vi "demoMode.vi"(8 "error in (no error)":errorcluster, 11 "Pod Drive in":refnum<class "Drive.lvclass">) -> (0 "error out":errorcluster, 3 "Pod Drive out":refnum<class "Drive.lvclass">)   [LabVIEW 2019, in "DriveOld.lvlib" / "Drive.lvclass"]
doc: "This VI puts the robot into demo mode. This will reduce the amount of power making the robot slower and safer."
uses:
  Drive.lvclass
  <vilib>/Rock Robotics/SystemInterfaces/DIO/FPGA_DIOChannel.ctl
  Drive.lvclass/Drive.ctl
  <vilib>/Rock Robotics/Network Tables/NT Write Boolean.vi
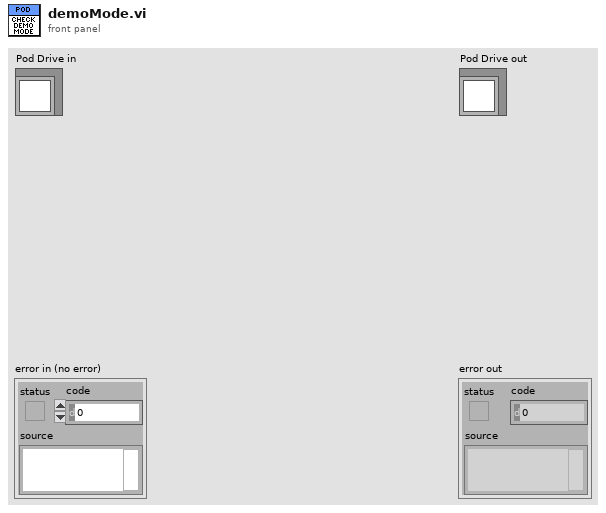
[diagram p1: front panel]
types:
  T1 = typedef "FPGA_DIOChannel.ctl" = enum8{"DIO 0", "DIO 1", "DIO 2", "DIO 3", "DIO 4", "DIO 5", "DIO 6", "DIO 7", "DIO 8", "DIO 9", "DIO MXP 0", "DIO MXP 1", "DIO MXP 2", "DIO MXP 3", "DIO MXP 4", "DIO MXP 5", "DIO MXP 6", "DIO MXP 7", "DIO MXP 8", "DIO MXP 9", "DIO MXP 10", "DIO MXP 11", "DIO MXP 12", "DIO MXP 13", "DIO MXP 14", "DIO MXP 15", "SPI Port CS1", "SPI Port CS2", "SPI Port CS3", "SPI Port MISO", "SPI Port MOSI", "Invalid"}
  T2 = typedef "WPI_DigitalInputDevRef.ctl" = cluster{"DevStatus":errorcluster, "DIO Channel":T1}
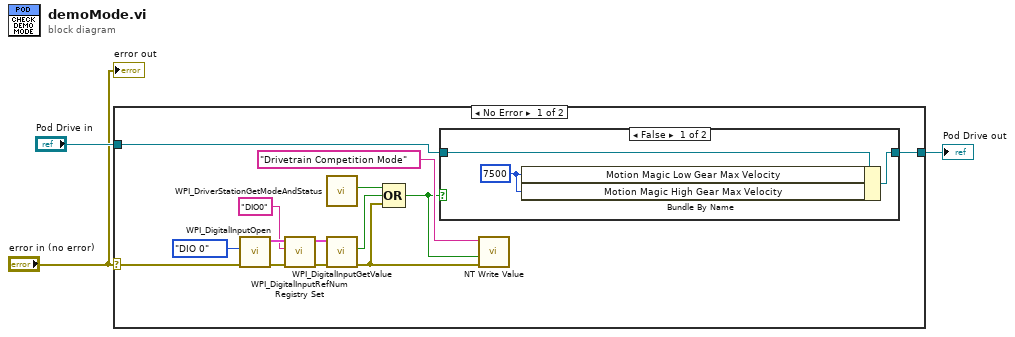
[diagram p0: block diagram]
diagram:
  n1 = case shown="No Error" "error in (no error)" {
    selector: "error in (no error)" -> [w5 _]
    tunnel: [w6 w22] -> w3
    tunnel: "Pod Drive in" -> [w7 w22]
    frame No Error {
      n2 = call <vilib>:"WPI_DigitalInputOpen.vi"("error in (no error)"=w5, "DIO Channel"=FPGA_DIOChannel."DIO 0") -> ("error out"=w16:errorcluster, "DigitalInputDevRef"=w15:T2)  [unwired: 8 in]
      n3 = call <vilib>:"WPI_DigitalInputRefNum Registry Set.vi"("error in (no error)"=w16, "refnum name"="DIO0", "DigitalInputDevRef"=w15) -> ("error out"=w13:errorcluster, "DigitalInputDevRef"=w12:T2)  [unwired: 7 in]
      n4 = call <vilib>:"WPI_DriverStationGetModeAndStatus.vi"() -> ("FMS Attached"=w9:bool)  [unwired: 10 in, 1 out]
      n5 = call <vilib>:"WPI_DigitalInputGetValue.vi"("error in (no error)"=w13, "DigitalInputDevRef"=w12) -> ("error out"=w4:errorcluster, "Value"=w11:bool)  [unwired: 7 in, 1 out]
      n6 = Compound Arithmetic op=OR(w9, w11, w4) -> (w8:bool)
      n7 = case shown="False" w8 {
        tunnel: w7 -> [w20 w21]
        tunnel: [w18 w21] -> w6
        frame False {
          w19 = u32 7500
          n8 = Bundle By Name(cluster=w20, "Motion Magic Low Gear Max Velocity"=w19, "Motion Magic High Gear Max Velocity"=w19) -> (w18:refnum<class "Drive.lvclass">)
        }
        frame True {
        }
      }
      n9 = call-poly <vilib>:"NT Write Value.vi"("error in"=w4, "Boolean"=w8, "Name"="Drivetrain Competition Mode") -> ()  [unwired: 8 in, 1 out]
    }
    frame Error {
    }
  }
  "Pod Drive out" <- w3
  "error out" <- "error in (no error)"
